vi "Launch Object by Type.vi"(8 "error in (no error)":errorcluster, 9 "Requestor":string, 10 "Type":string, 11 "Application Controller in":refnum<class "Application Controller.lvclass">) -> (0 "error out":errorcluster, 3 "Application Controller out":refnum<class "Application Controller.lvclass">)   [LabVIEW 2016, in "Application Controller.lvclass"]
uses:
  Application Controller.lvclass
  Template Module/Template Module.lvclass
  Application Controller.lvclass/Application Controller.ctl
  Template Module Messages/Launch Object by Type Response Msg/Launch Object by Type Response Msg.lvclass/Launch Object by Type Response Msg.ctl
  <vilib>/ActorFramework/Message Enqueuer/Message Enqueuer.lvclass/Message Enqueuer.ctl
  <vilib>/ActorFramework/Message Enqueuer/Enqueue.vi
  Template Module Messages/Launch Object by Type Response Msg/Launch Object by Type Response Msg.lvclass
  C:/Program Files/National Instruments/LabVIEW 2016/vi.lib/ActorFramework/Message/Message.lvclass
  <vilib>/ActorFramework/Message Priority Queue/Priority Enqueue.vi
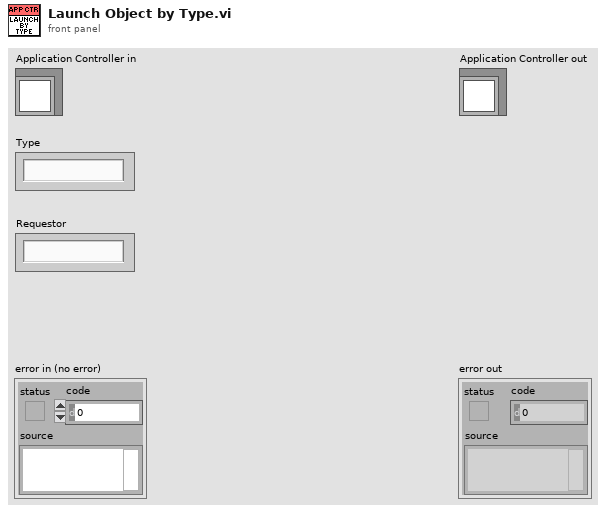
[diagram p1: front panel]
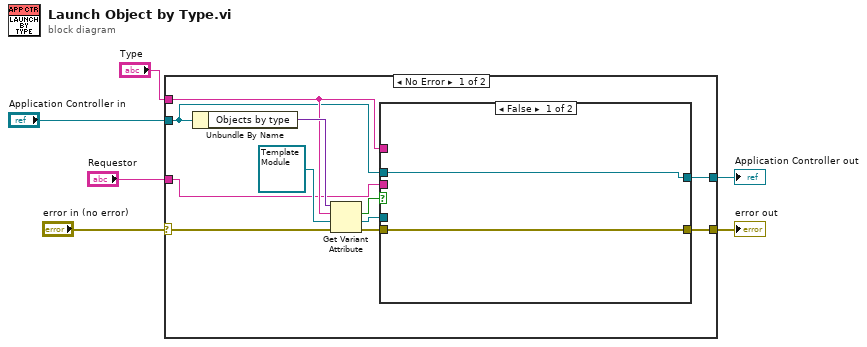
[diagram p0: block diagram]
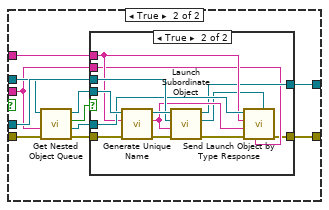
[diagram p2: hidden frame]
diagram:
  n1 = case shown="No Error" "error in (no error)" {
    selector: "error in (no error)" -> [w8 w47]
    tunnel: [w7 w47] -> w5
    tunnel: [w9 w46] -> w3
    tunnel: "Application Controller in" -> [w10 w46]
    tunnel: "Type" -> [w14 _]
    tunnel: "Requestor" -> [w11 _]
    frame No Error {
      n2 = Unbundle By Name(w10) -> ("Objects by type"=w17:variant)
      n3 = Get Variant Attribute(Variant=w17, name=w14, default value (empty Variant)=refnum<class "Template Module.lvclass"> refnum ("Da Base.lvclass"), error in=w8) -> (found=w15:bool, value=w13:refnum<class "Template Module.lvclass">, error out=w12:errorcluster)  [unwired: 1 out]
      n4 = case shown="False" w15 {
        tunnel: w10 -> [w19 w29]
        tunnel: w14 -> [_ w21]
        tunnel: w13 -> [_ w30]
        tunnel: w12 -> [w18 w27]
        tunnel: w11 -> [_ w20]
        tunnel: [w19 w23] -> w9
        tunnel: [w18 w22] -> w7
        frame False {
        }
        frame True {
          n5 = call-dynamic "Get Nested Object Queue.vi"("error in (no error)"=w27, "Name"=w20, "Measure Object in"=w29) -> ("error out"=w26:errorcluster, "Object Enqueuer"=w24:refnum<class "Message Enqueuer.lvclass">, "Found?"=w28:bool, "Measure Object out"=w25:refnum<class "Application Controller.lvclass">)  [unwired: 5 in]
          n6 = case shown="True" w28 {
            tunnel: w21 -> [_ w39]
            tunnel: w30 -> [_ w44]
            tunnel: w26 -> [w31 w42]
            tunnel: w25 -> [w32 w41]
            tunnel: w24 -> [_ w40]
            tunnel: [w32 w36] -> w23
            tunnel: [w31 w34] -> w22
            tunnel: w20 -> [_ w35]
            frame False {
            }
            frame True {
              n7 = call-dynamic "Generate Unique Name.vi"("error in (no error)"=w42, "Type"=w39, "Da Base in"=w41) -> ("error out"=w43:errorcluster, "Unique name"=w38:string, "Da Base out"=w45:refnum<class "Application Controller.lvclass">)  [unwired: 6 in]
              n8 = call-dynamic "Launch Subordinate Object.vi"("error in (no error)"=w43, "Name"=w38, "Subordinate Object"=w44, "Measure Object in"=w45) -> ("error out"=w37:errorcluster, "Nested Actor's Enqueuer"=w33:refnum<class "Message Enqueuer.lvclass">, "Measure Object out"=w36:refnum<class "Application Controller.lvclass">)  [unwired: 5 in]
              n9 = call "Send Launch Object by Type Response.vi"("Enqueuer"=w33, "Requestor"=w35, "error in (no error)"=w37, "Name"=w38, "Type"=w39, "Message Enqueuer"=w40) -> ("error out"=w34:errorcluster)  [unwired: 4 in, 1 out]
            }
          }
        }
      }
    }
    frame Error {
    }
  }
  "error out" <- w5
  "Application Controller out" <- w3
